vi "Write Results.vi"(9 "Analyze Results Fluence.lvclass":refnum<class "Analyze Results Fluence.lvclass">, 10 "Analyze Results Energy Obj":refnum<class "Analyze Results Energy.lvclass">, 11 "Analyze Results Fluence and Energy in":refnum<class "Analyze Results Fluence and Energy.lvclass">) -> (3 "Analyze Results Fluence and Energy out":refnum<class "Analyze Results Fluence and Energy.lvclass">)   [LabVIEW 2014, in "Analyze Results Fluence and Energy.lvclass"]
doc: "Hier werden nur die Physikalische Ergebnise übergeben. Die Einstellungen zu Overlays bleiben unverändert."
uses:
  Analyze Results Fluence and Energy.lvclass
  JETI200 Overview and ShotID/HIJ Vision/Analyze/Results and Overlays/Results Energy/Analyze Results Energy.lvclass
  JETI200 Overview and ShotID/HIJ Vision/Analyze/Results and Overlays/Results Fluence/Analyze Results Fluence.lvclass
  JETI200 Overview and ShotID/HIJ Vision/Analyze/Results and Overlays/Results Energy/Analyze Results Energy.lvclass/Analyze Results Energy.ctl
  Analyze Results Fluence and Energy.lvclass/Analyze Results Fluence and Energy.ctl
  JETI200 Overview and ShotID/HIJ Vision/Analyze/Results and Overlays/Results Energy/Write Energy.vi
  JETI200 Overview and ShotID/HIJ Vision/Analyze/Results and Overlays/Results Energy/Read Energy.vi
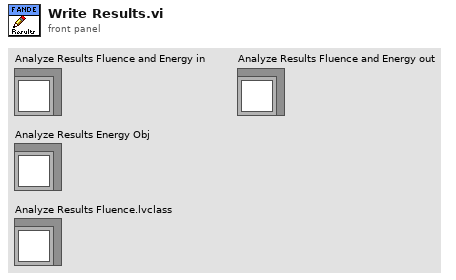
[diagram p1: front panel]
types:
  T1 = typedef "Analyze.lvlib/Analyze Fluence.lvclass/Fluence Info.ctl" = cluster{"Fluence J/cm^2":dbl[unit], "Energy in Area":dbl[unit], "max value":i64, "Max fluence area":cluster{"Left":i32, "Top":i32, "Right":i32, "Bottom":i32}}
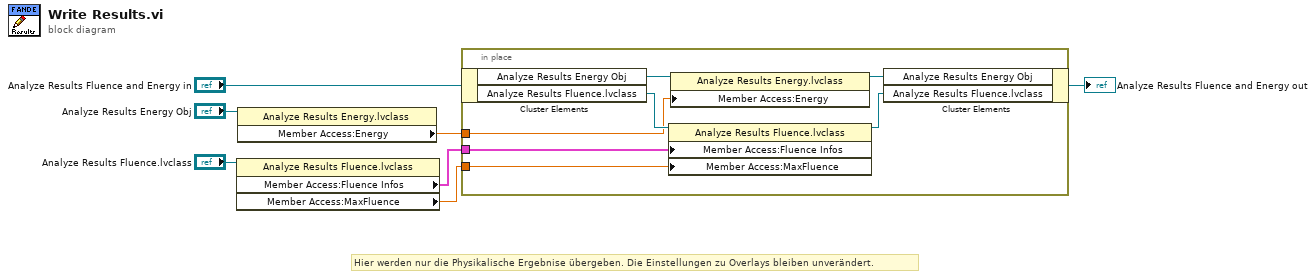
[diagram p0: block diagram]
diagram:
  # "Hier werden nur die Physikalische Ergebnise übergeben. Die Einstellungen zu Overlays bleiben unverändert."
  n1 = property class="Analyze Results Fluence.lvclass"(reference="Analyze Results Fluence.lvclass") -> ("Member Access:Fluence Infos"=w2:T1[], "Member Access:MaxFluence"=w1:dbl[unit])  [unwired: 1 in, 2 out]
  n2 = property class="Analyze Results Energy.lvclass"(reference="Analyze Results Energy Obj") -> ("Member Access:Energy"=w3:dbl[unit])  [unwired: 1 in, 2 out]
  n3 = in-place {
    in-place-border: w3 -> [w10]
    in-place-border: w2 -> [w9]
    in-place-border: w1 -> [w8]
    n4 = in-place-cluster #1("Analyze Results Fluence and Energy in") -> ("Analyze Results Energy Obj"=w14:refnum<class "Analyze Results Energy.lvclass">, "Analyze Results Fluence.lvclass"=w13:refnum<class "Analyze Results Fluence.lvclass">)
    n5 = property class="Analyze Results Fluence.lvclass"(reference=w13, "Member Access:Fluence Infos"=w9, "Member Access:MaxFluence"=w8) -> (reference out=w11:refnum<class "Analyze Results Fluence.lvclass">)  [unwired: 1 in, 1 out]
    n6 = property class="Analyze Results Energy.lvclass"(reference=w14, "Member Access:Energy"=w10) -> (reference out=w12:refnum<class "Analyze Results Energy.lvclass">)  [unwired: 1 in, 1 out]
    n7 = in-place-cluster #1("Analyze Results Energy Obj"=w12, "Analyze Results Fluence.lvclass"=w11) -> (→"Analyze Results Fluence and Energy out":refnum<class "Analyze Results Fluence and Energy.lvclass">)
  }
